vi "dbc-to-tree.vi"(8 "error in (no error)":errorcluster, 11 "dbc in":refnum<class "dbc.lvclass">) -> (0 "error out":errorcluster, 3 "dbc out":refnum<class "dbc.lvclass">)   [LabVIEW 2015, in "dbc.lvclass"]
uses:
  dbc.lvclass
  dbc.lvclass/dbc.ctl
  read-tree-ref.vi
  read-file-data.vi
  read-dbc-content.vi
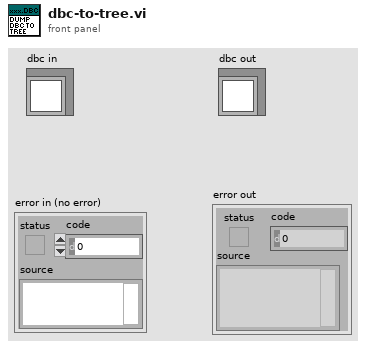
[diagram p1: front panel]
types:
  T1 = typedef "dbc-file-data.ctl" = cluster{"dbc.ref":refnum<k21>, "dbc.file":path, "alias":string}
  T2 = typedef "dbc-content-data.ctl" = cluster{"Number of Clusters":i32, "Number of Frames ":i32[], "Clusters":string[], "Frames":string[][], "Signals":string[][][], "Number of Signals":i32[][]}
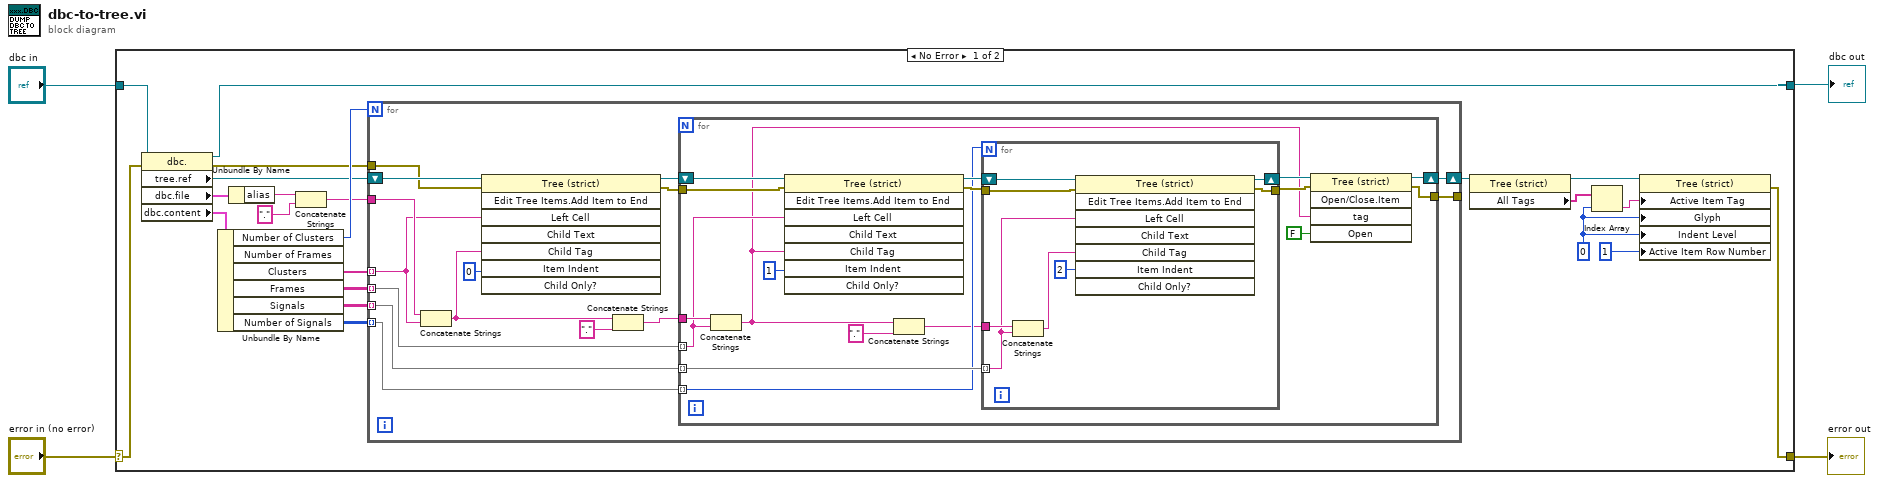
[diagram p0: block diagram]
diagram:
  n1 = case shown="No Error" "error in (no error)" {
    selector: "error in (no error)" -> [w14 w68]
    tunnel: [w11 w68] -> w3
    tunnel: [w13 w67] -> w1
    tunnel: "dbc in" -> [w26 w67]
    frame No Error {
      w6 = 0
      n2 = property class="dbc."(reference=w26, error in=w14) -> (reference out=w13:refnum<class "dbc.lvclass">, error out=w10:errorcluster, "tree.ref"=w23:refnum<vi>, "dbc.file"=w21:T1, "dbc.content"=w25:T2)
      n3 = Unbundle By Name(w25) -> ("Number of Clusters"=w24:i32, "Clusters"=w22:string[], "Frames"=w17:string[][], "Signals"=w16:string[][][], "Number of Signals"=w15:i32[][])  [unwired: 1 out]
      n4 = Unbundle By Name(w21) -> ("alias"=w20:string)
      n5 = Concatenate Strings(w20, "." ("string")) -> (w18:string)
      n6 = for {
        N: w24 -> [_]
        shift-right: [w37] -> w12
        shift-left: w23 -> [w41]
        tunnel: w22 -> [w39] mode=indexing
        tunnel: w18 -> [w40]
        tunnel: w17 -> [w36] mode=indexing
        tunnel: w16 -> [w35] mode=indexing
        tunnel: w10 -> [w33]
        tunnel: w15 -> [w32] mode=indexing
        tunnel: [w31] -> _
        n7 = Concatenate Strings(w40, w39) -> (w27:string)
        n8 = invoke class="Tree (strict)" method="Edit Tree Items.Add Item to End"(reference=w41, error in=w33, "Left Cell"=w39, "Child Tag"=w27, "Item Indent"=0 ("New Item Indentation")) -> (reference out=w38:refnum<vi>, error out=w34:errorcluster)  [unwired: 3 in, 6 out]
        n9 = Concatenate Strings(w27, "." ("string")) -> (w30:string)
        n10 = for {
          shift-right: [w43] -> w37
          shift-left: w38 -> [w58]
          tunnel: w36 -> [w48] mode=indexing
          tunnel: w35 -> [w55] mode=indexing
          tunnel: w34 -> [w54]
          tunnel: w32 -> [w52] mode=indexing
          tunnel: [w42] -> w31
          tunnel: w30 -> [w49]
          n11 = Concatenate Strings(w49, w48) -> (w45:string)
          n12 = invoke class="Tree (strict)" method="Edit Tree Items.Add Item to End"(reference=w58, error in=w54, "Left Cell"=w48, "Child Tag"=w45, "Item Indent"=1 ("New Item Indentation")) -> (reference out=w57:refnum<vi>, error out=w53:errorcluster)  [unwired: 3 in, 6 out]
          n13 = Concatenate Strings(w45, "." ("string")) -> (w47:string)
          n14 = for {
            N: w52 -> [_]
            shift-right: [w65] -> w56
            shift-left: w57 -> [w66]
            tunnel: w55 -> [w60] mode=indexing
            tunnel: w53 -> [w63]
            tunnel: [w62] -> w51
            tunnel: w47 -> [w61]
            n15 = Concatenate Strings(w61, w60) -> (w59:string)
            n16 = invoke class="Tree (strict)" method="Edit Tree Items.Add Item to End"(reference=w66, error in=w63, "Left Cell"=w60, "Child Tag"=w59, "Item Indent"=2 ("New Item Indentation")) -> (reference out=w65:refnum<vi>, error out=w62:errorcluster)  [unwired: 3 in, 6 out]
          }
          n17 = invoke class="Tree (strict)" method="Open/Close.Item"(reference=w56, error in=w51, "tag"=w45, "Open"=FALSE ("Open?")) -> (reference out=w43:refnum<vi>, error out=w42:errorcluster)  [unwired: 1 in, 3 out]
        }
      }
      n18 = property class="Tree (strict)"(reference=w12) -> (reference out=w9:refnum<vi>, "All Tags"=w8:string[])  [unwired: 1 in, 1 out]
      n19 = Index Array(array=w8, index=w6) -> (element=w7:string)
      n20 = property class="Tree (strict)"(reference=w9, "Active Item Tag"=w7, "Glyph"=w6, "Indent Level"=w6, "Active Item Row Number"=1 ("Active Item:Row Number")) -> (error out=w11:errorcluster)  [unwired: 1 in, 1 out]
    }
    frame Error {
    }
  }
  "error out" <- w3
  "dbc out" <- w1
